vi "Tree Clear.vi"(8 "error in (no error)":errorcluster, 11 "[V]System Tree View in":refnum<class "[V]System Tree View.lvclass">) -> (0 "error out":errorcluster, 3 "[V]System Tree View out":refnum<class "[V]System Tree View.lvclass">)   [LabVIEW 2020, in "[V]System Tree View.lvlib" / "[V]System Tree View.lvclass"]
uses:
  [V]System Tree View.lvclass
  [V]System Tree View.lvclass/[V]System Tree View.ctl
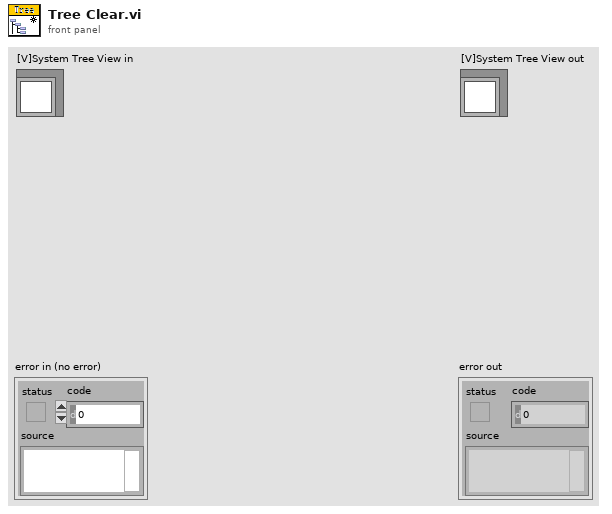
[diagram p1: front panel]
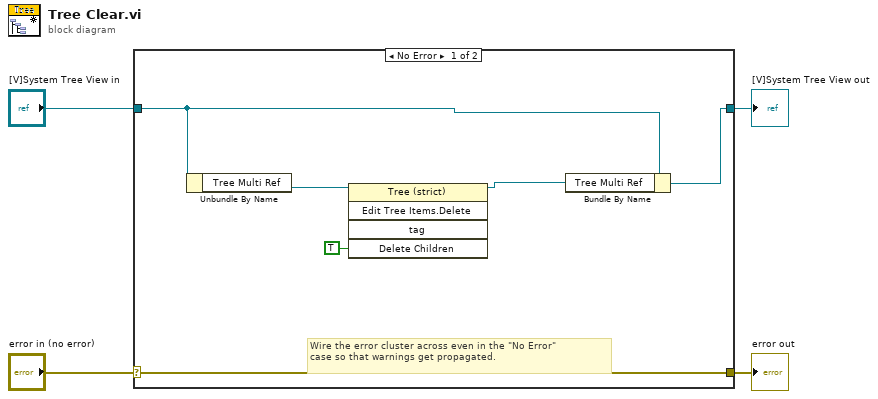
[diagram p0: block diagram]
diagram:
  n1 = case shown="No Error" "error in (no error)" {
    selector: "error in (no error)" -> [w10 w12]
    tunnel: [w10 w12] -> w3
    tunnel: [w5 w11] -> w1
    tunnel: "[V]System Tree View in" -> [w7 w11]
    frame No Error {
      # "Wire the error cluster across even in the \"No Error\"\ncase so that warnings get propagated."
      n2 = Unbundle By Name(w7) -> ("Tree Multi Ref"=w8:refnum<vi>)
      n3 = invoke class="Tree (strict)" method="Edit Tree Items.Delete"(reference=w8, "Delete Children"=TRUE ("Delete Children?")) -> (reference out=w6:refnum<vi>)  [unwired: 3 in, 4 out]
      n4 = Bundle By Name(cluster=w7, "Tree Multi Ref"=w6) -> (w5:refnum<class "[V]System Tree View.lvclass">)
    }
    frame Error {
    }
  }
  "error out" <- w3
  "[V]System Tree View out" <- w1
